vi "设置字体.vi"(8 "error in (no error)":errorcluster caption="错误输入（无错误）", 11 "程序 输入":refnum<class "程序.lvclass">) -> (0 "error out":errorcluster caption="错误输出", 3 "程序 输出":refnum<class "程序.lvclass">)   [LabVIEW 2018, in "程序.lvclass"]
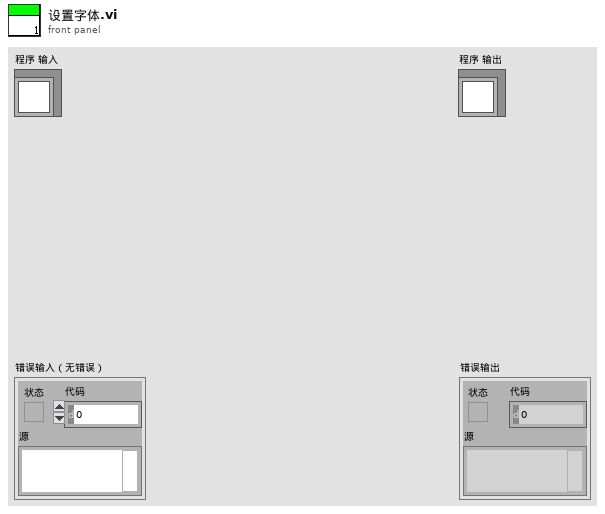
[diagram p1: front panel]
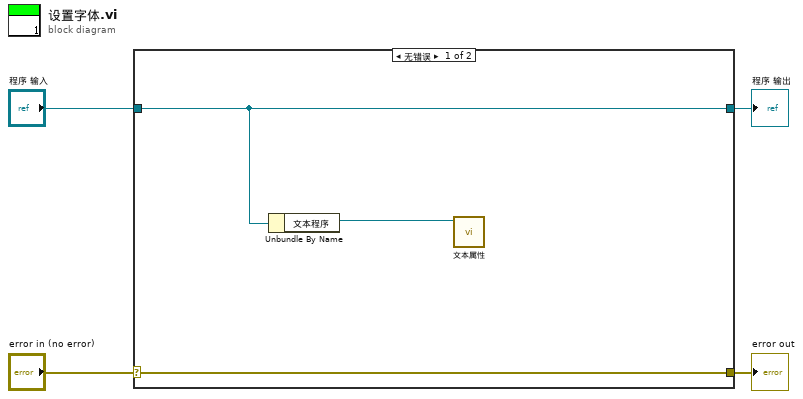
[diagram p0: block diagram]
diagram:
  n1 = case shown="无错误" "error in (no error)" {
    selector: "error in (no error)" -> [w7 w9]
    tunnel: [w7 w9] -> w3
    tunnel: [w6 w8] -> w1
    tunnel: "程序 输入" -> [w6 w8]
    frame No Error {
      n2 = Unbundle By Name(w6) -> ("文本程序"=w5:refnum<vi>)
      n3 = call "文本属性.vi"("引用"=w5) -> ()  [unwired: 11 in]
    }
    frame Error {
    }
  }
  "error out" <- w3
  "程序 输出" <- w1
